vi "output.vi"(8 "error in":errorcluster, 10 "output data":T1, 11 "module in":refnum<class "E2E Runtime (UDP).lvclass">) -> (0 "error out":errorcluster, 2 "output allocation":T1, 3 "module out":refnum<class "E2E Runtime (UDP).lvclass">)   [LabVIEW 2015, in "E2E Runtime (UDP).lvclass"]
doc: "Provides an interface for writing data to a module at runtime. While this interface performs no operations, a child should provide an override which may write to any open sessions, references, or interfaces."
uses:
  E2E Runtime (UDP).lvclass
  <vilib>/NI/Tag Bus/table/data table.ctl
  E2E Runtime (UDP).lvclass/E2E Runtime (UDP).ctl
  <vilib>/NI/Tag Bus/table/data table.lvlib
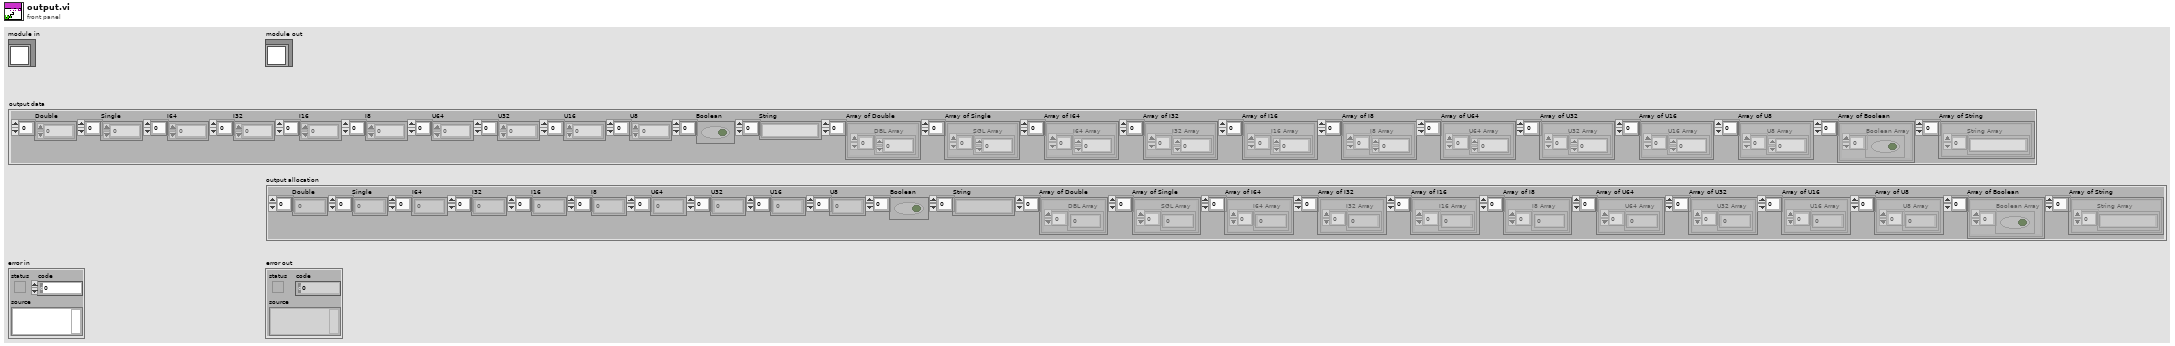
[diagram p1: front panel]
types:
  T1 = typedef "tag bus.lvlib/data table.lvlib/data table.ctl" = cluster{"Double":dbl[], "Single":sgl[], "I64":i64[], "I32":i32[], "I16":i16[], "I8":i8[], "U64":u64[], "U32":u32[], "U16":u16[], "U8":u8[], "Boolean":bool[], "String":string[], "Array of Double":cluster{"DBL Array":dbl[]}[], "Array of Single":cluster{"SGL Array":sgl[]}[], "Array of I64":cluster{"I64 Array":i64[]}[], "Array of I32":cluster{"I32 Array":i32[]}[], "Array of I16":cluster{"I16 Array":i16[]}[], "Array of I8":cluster{"I8 Array":i8[]}[], "Array of U64":cluster{"U64 Array":u64[]}[], "Array of U32":cluster{"U32 Array":u32[]}[], "Array of U16":cluster{"U16 Array":u16[]}[], "Array of U8":cluster{"U8 Array":u8[]}[], "Array of Boolean":cluster{"Boolean Array":bool[]}[], "Array of String":cluster{"String Array":string[]}[]}
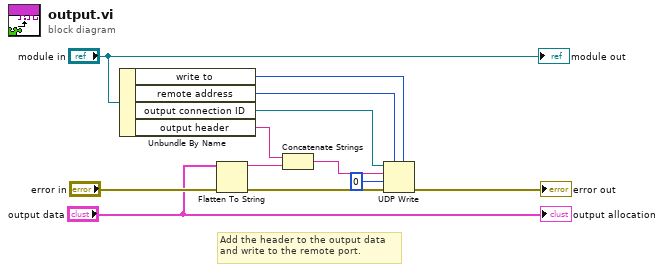
[diagram p0: block diagram]
diagram:
  # "Add the header to the output data\nand write to the remote port."
  n1 = Unbundle By Name("module in") -> ("write to"=w8:u16, "remote address"=w9:u32, "output connection ID"=w10:refnum<k16>, "output header"=w5:string)
  n2 = Flatten To String(anything="output data", error in (no error)="error in") -> (data string=w6:string, error out=w3:errorcluster)  [unwired: 2 in, 1 out]
  n3 = Concatenate Strings(w5, w6) -> (w4:string)
  n4 = UDP Write(address=w9, port or service name=w8, connection ID=w10, data in=w4, 8:w3, 9:0 ("timeout ms (25000)")) -> (error out=→"error out":errorcluster)  [unwired: 1 out]
  "module out" <- "module in"
  "output allocation" <- "output data"
